vi "MsgSaveTracepoints.vi"() -> (1 "message name":string)   [LabVIEW 2017, in "TraceLogger.lvlib"]
uses:
  <vilib>/addons/TraceLogger/TraceLogger.lvlib
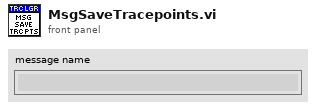
[diagram p1: front panel]
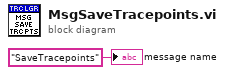
[diagram p0: block diagram]
diagram:
  "message name" <- "SaveTracepoints" ("ProcessName")
